vi "Main-dataQ.vi"() -> ()   [LabVIEW 2013]
uses:
  ctl/config_ctl.ctl
  ctl/strain_ctl.ctl
  <vilib>/measure/mascope.llb/Amplitude and Levels 1 chan.vi
  <vilib>/measure/NI_MAPro.lvlib
panel:
  out "error out":errorcluster
  out "원소":enum16{"ini", "grab", "close"}(ring)
  out "grab loop":i32
  out "cam loop":i32
  out "strain loop":i32
  in  "Nulling":bool
  in  "pause":bool
  in  "START":bool
  in  "save_setting":bool
  in  "load_setting":bool
  out "data loop":i32
  out "dt":u32
  in  "Main tap":T1(tab)
  out "right":dbl(slide) scale=0.0..0.5
  out "left":dbl(slide)
  out "rear":dbl(slide) scale=0.0..0.5
  out "front":dbl(slide)
  out "trigger":bool
  out "Triggered Force graph":waveform(dbl)(graph)={"t0"=timestamp(0 s since 1904-01-01), "dt"=0.00062, "Y"=array[3100 elements]}
  out "bonding force":dbl=1.1386680148675508 caption="Bonding force (kg)" format="%.3f"
  out "Bonding time":dbl=0.5053000000000001 format="%.3f"
  out "vacum":dbl=1.2177873383633695 format="%#_3f"
  out "Heater temp":dbl=nan format="%0.2f"
  out "XY 그래프":cluster{dbl[], dbl[]}(graph)
  out "Filtered force 그래프":waveform(dbl)[](graph)
  out "vacuum 차트 3":waveform(dbl)(graph)={"t0"=timestamp(3477442777.176875 s since 1904-01-01), "dt"=0.01, "Y"=[0.9261417940939543, 0.9261417940939543, 0.9261417940939543, 0.9261417940939543, 0.9261417940939543, 0.9261417940939543, 0.9261417940939543, 0.9261417940939543, 0.9261417940939543, 0.9261417940939543], "attributes"=variant("NI_ChannelName"=variant(string "전압"), "NI_UnitDescription"=variant(string "Volts"))}
  out "Force raw chart":waveform(dbl)[](graph)=[{"t0"=timestamp(3477442777.13187 s since 1904-01-01), "dt"=0.00062, "Y"=[-1.6112136636470233e-05, -8.569886798010926e-06, -1.9875060209823524e-07, 2.38297423695265e-06, -2.5658168581669667e-06, -1.772821098699811e-06, -4.127955201515539e-06, 6.359857628775875e-07, 4.928880013384412e-07, -3.030881455329775e-06, -1.6476111269731543e-06, -3.5257574105908386e-06, 3.9272455815972755e-06, 4.1657435117466915e-06, 1.9357923056845556e-06, -8.873963893666015e-06, -7.478785108954976e-06, 2.961286460921625e-07, 1.4110617831093333e-07, -1.8980310390713461e-06, 1.6734457588159683e-06, -1.091306434532689e-05, -1.0513727362142483e-06, -6.190924313818898e-06, -1.2540761368932031e-05, -2.1656959207560037e-05, -7.4907097304474685e-06, -3.2872630354662113e-06, -7.950263527933837e-08, -5.964355867846931e-06, -2.4107952296524134e-06, -3.7881010918357573e-06, 2.609546568115507e-06, 1.715182700246618e-06, -5.290612250873919e-06, -6.512889823589868e-06, -3.120361442334684e-07, 5.578846081749961e-06, 7.045614998740958e-06, -1.4627773018794912e-06, -7.937882831116044e-06, -2.595628704294203e-06, 1.2799261966089874e-06, 3.3190306855961753e-07, -3.4363220332503078e-06, -9.953137975658443e-06, 2.3591245238553327e-06, -1.0871470597100204e-06, 8.685197127258367e-07, -7.478785108954976e-06, -8.659321257106097e-06, -4.879210834785539e-06, -3.710590473067321e-06, -4.771888670569855e-06, -1.2516912366543758e-05, -5.576804340679935e-06, -6.274396873296863e-06, -8.546139112344271e-07, 2.2696881098723825e-06, -3.585380986597095e-06, -7.890184386099151e-06, 4.034519211733817e-07, 2.055040781583931e-06, 3.3071514956147953e-06, -2.7625750097582926e-06, -6.900440625190667e-06, 4.2909549706155075e-06, 9.830102788370948e-06, 3.032879356729265e-06, 4.088231671969834e-06, -9.488079817087242e-06, -5.111742111559042e-06, 2.567809552028929e-06, -4.688415860253707e-06, -1.833603522524735e-05, -9.50012139076079e-07, 3.3250388142463035e-06, -2.6135158111173114e-06, -6.769269618278701e-06, -2.0929577385222132e-05, -7.305878065355784e-06, -1.8562943957647073e-06, -3.090505090348801e-06, -3.5257574105908386e-06, -4.932871908254762e-06, -1.033522309183479e-07, -4.169691655199052e-06, 1.94771715199473e-06, -5.254838228130094e-06, -5.147516144541169e-06, 1.2978134427175586e-06, 9.126526251121246e-06, 1.5422725370008507e-06, -4.688415860253707e-06, -2.005353820147982e-06, 4.4518875659287035e-07, 1.7688444872052448e-06, -1.1229213806461855e-06, -6.51885214588969e-06, -1.4490413466475015e-05], "attributes"=variant("NI_ChannelName"=variant(string "변형률_0"), "NI_UnitDescription"=variant(string "Strain"))}, {"t0"=timestamp(3477442777.13187 s since 1904-01-01), "dt"=0.00062, "Y"=[-1.5926450874775857e-06, 1.7934307923881257e-06, -2.236473822173629e-06, -4.09045749208906e-06, -3.881810155491518e-06, 1.7218937409129746e-06, 3.9872386740088464e-06, 1.7192680555871353e-07, 2.2286147427125606e-06, -1.3005373326004466e-06, 3.456670124526979e-06, 8.523920832607e-06, 5.322604705970085e-06, 3.104945216654824e-06, 2.639953345335169e-06, 6.449322569493326e-06, 1.898110120282012e-07, -2.9306233811443237e-07, -7.929552945691535e-06, 2.53892933758521e-05, 6.6698972632327115e-06, 5.113953528386892e-06, 2.425341858268832e-06, -5.911320745626876e-07, -2.8385721664852527e-06, 1.0303694376600552e-06, -3.2286931975534613e-07, -4.793896442446842e-06, -2.7789585013682837e-06, -2.254357941858881e-06, 4.482039064584e-06, 3.188405341896096e-06, 2.890333530003795e-06, 1.5370897386411374e-06, 1.3224787249476363e-06, 5.0603003825103886e-06, 4.470116157849115e-06, 2.0378491288205883e-06, 3.087060905915481e-06, 4.237619533343155e-06, 6.22874797305966e-06, 2.4551490037417866e-06, 8.455656909807571e-07, -1.976799849226179e-07, -2.862417630541878e-06, 5.030493081733363e-06, 2.8068734545164028e-06, -7.640124402846258e-07, -2.105323591603382e-06, 2.3750223240719277e-07, 6.884510572159387e-06, -7.878580032793122e-07, -5.163499562134611e-06, -6.391533772034915e-06, -2.6835766223972933e-06, 4.684728522578421e-06, 2.885317683250044e-08, -1.2826531787987904e-06, -2.8206880676963555e-06, 3.7726266086577194e-06, 6.7414350226397595e-06, 3.3195569954219583e-06, 2.017338166964026e-07, 2.7114905281608864e-06, 3.40301715648635e-06, 9.60891530636603e-06, -7.029395011258529e-06, 2.153804825353152e-05, 1.1194680695472973e-05, -9.786224662971449e-07, 8.702765913475292e-06, -2.558387878634849e-06, -5.911320745626876e-07, -2.4272377325028147e-06, 2.8307191889483254e-06, 5.656446771208991e-06, 1.9901577367198323e-06, -2.2960875519699664e-06, -4.656785538247539e-06, -2.898185824494624e-06, 7.501831387741804e-07, -3.983153158427838e-06, -1.610529230191517e-06, -2.8028039682679484e-06, 4.458193251398366e-06, 9.171026170763248e-07, 3.748780829304955e-06, 1.9577241432685033e-07, 3.206289656260379e-06, 2.0974633753433343e-06, 7.442217298655735e-07, 6.548006047634227e-07, -1.8489844052503307e-06, 3.7964723891478954e-06, 8.0470009297029e-06, 2.5863004649327575e-06, 1.1674819390124968e-06, 3.150004752252312e-07, 3.188405341896096e-06, 5.7637531966593845e-06], "attributes"=variant("NI_ChannelName"=variant(string "변형률_1"), "NI_UnitDescription"=variant(string "Strain"))}, {"t0"=timestamp(3477442777.13187 s since 1904-01-01), "dt"=0.00062, "Y"=[-9.774144215970737e-06, -5.761376757146625e-06, 5.947220028941115e-07, -3.8056626676763385e-06, -7.275857412313684e-06, 3.1765375395588494e-06, -3.1557437920494864e-06, -3.000717146469372e-06, 7.974506851273759e-07, -1.8618660842482212e-06, -1.4862235419361472e-06, -6.721343374039278e-06, 8.62045556081355e-06, -3.294812422418737e-07, 2.115189123215763e-06, -2.3030966465335333e-06, -5.773301819593379e-06, -1.1940569250260916e-06, -5.171085810533189e-06, -2.538875015539028e-08, 3.6814298472928053e-07, -8.939395837287375e-06, 2.401395215885246e-06, -4.646382161832467e-06, -7.311632490439199e-06, -2.205074690463858e-05, -3.5313850800753163e-06, -4.425767963291082e-06, -3.6148608835335274e-06, -1.677026138378287e-06, -2.5952626153941553e-06, 3.26404755740087e-07, -2.601225184409818e-06, 1.4056372250135049e-06, -1.1753684800069817e-05, -4.914696596438629e-06, 5.808765257422834e-08, 6.318857576908811e-06, 3.9934195965366175e-06, 5.03688401927312e-06, -6.059503232998047e-06, -5.4811377077647035e-06, 1.3937119916306282e-06, -7.055244373975443e-06, 7.318619848217363e-07, -1.718764196644247e-06, 4.814324809771893e-07, -1.0119968136008337e-05, 1.984011385493666e-06, -1.0131893094502119e-05, -1.0251142663796572e-05, -3.865288210289022e-06, -6.06546576070178e-06, -6.995619211769368e-06, 2.1867406310243084e-06, -1.0119968136008337e-05, -8.080796051007461e-06, -1.7962777241804084e-06, -1.2536827790775241e-06, 1.4771886312832808e-06, 2.2284790153078483e-06, -6.190678826058288e-06, -1.7068390374955085e-06, 1.4593007787556523e-06, 5.024958699283277e-06, 2.1927032571370627e-06, 5.589463616211063e-07, -4.831221009990731e-06, -8.959275481128778e-07, 3.421005752440379e-06, 3.987456948949547e-06, -4.205153667407975e-06, -9.674786147839707e-07, -5.212823577128643e-06, -1.6183772832057885e-05, 9.294241431321112e-06, -3.257107342016943e-06, -4.473468338791205e-06, -1.0316729914785664e-05, -1.128265025116678e-05, -1.0650628513704086e-05, -4.65234470638786e-06, -2.362722368329657e-06, -7.230124280525015e-07, 7.139741589589915e-07, -2.326946936105031e-06, -1.5277486145651072e-05, 1.411599841811428e-06, -3.3703959911923048e-06, -5.7852268817560655e-06, 2.17481537901177e-06, 2.5325730631100896e-06, -1.981117625965015e-06, -2.3209843638189005e-06, -2.6191128910294843e-06, 9.047776678219688e-07, -6.514613263977364e-07, -9.495908490762017e-07, 5.470211484321648e-07, -1.2970025127066287e-05], "attributes"=variant("NI_ChannelName"=variant(string "변형률_2"), "NI_UnitDescription"=variant(string "Strain"))}, {"t0"=timestamp(3477442777.13187 s since 1904-01-01), "dt"=0.00062, "Y"=[-7.598292136517871e-06, -3.990960943167142e-06, -3.961148180242939e-06, 8.446924425047726e-07, -3.865747326939833e-06, -6.459578537381319e-07, -5.028556181360945e-07, -4.313044849763774e-07, -2.0352399287900154e-06, -2.1843042998043006e-06, 2.317459299605134e-06, 2.520188680335006e-06, 1.8642998046072807e-06, 3.1998303138911986e-07, -2.3810692014959805e-06, 1.1129194138591358e-07, -3.919410309162601e-06, -4.181762583788524e-06, -2.9177003579997263e-06, -2.887887531081505e-06, 8.147893563887326e-08, -5.910899132064934e-06, 5.841384650575335e-06, -7.771348670609545e-07, -9.965402760758176e-06, -5.064219224553743e-06, -1.0078689889986319e-05, -8.14684269941332e-06, -4.8913055460130025e-06, -2.0292773530250545e-06, -2.5003206193811262e-06, -4.098286874975869e-06, -3.305266946174274e-06, -4.038661360148547e-06, -2.4228072009909966e-06, -2.1366037059148034e-06, -4.217537883299131e-06, -1.2183663865814867e-06, -2.5062831895288145e-06, 1.1725454274867201e-07, 3.9571845882479464e-06, -1.8087543828407676e-07, -4.0803992212742764e-06, -1.2064412154978175e-06, -5.839348772806825e-06, -1.8563626249113895e-06, -5.213282692541838e-06, -3.1800531582297593e-06, -1.8742503581789873e-06, -3.8360372384809986e-07, -4.181762583788524e-06, -6.0420747641119605e-06, -4.050586463682811e-06, -3.531844197032469e-06, -2.3452937705841765e-06, -7.1034036122986465e-06, -1.32569291353597e-06, -1.6953729967054738e-06, -1.7549987909737935e-06, -2.8699998340773e-06, -4.825717583337447e-06, -2.46454519700197e-06, 1.1964865605783791e-06, 3.378708431566748e-07, 2.889871880335409e-06, 2.0908795007679327e-06, -1.0514139655274806e-06, 5.501512595474361e-06, -3.376817668063878e-06, -4.819755040849376e-06, -1.5701588055974375e-06, -5.064219224553743e-06, -8.904240781442745e-07, 4.028736359651292e-06, -4.1996502338637966e-06, -6.918565604118794e-06, -3.996923495538705e-06, -3.3648925484600175e-06, -1.3024146240405366e-05, -8.289942747279497e-06, -7.061666003521132e-06, -5.165582387620764e-06, -6.823165315097408e-06, -1.0633391403086943e-06, -1.9517638616103747e-06, -5.255020455614867e-06, -2.4705077675762867e-06, -1.7491284040547266e-07, -3.1919782822420984e-06, -2.858074702385669e-06, -1.9815767443457687e-06, 2.317459299605134e-06, 3.927371353185168e-06, 3.665014961285459e-06, 2.186281508816372e-06, -1.0096758515535991e-06, -1.5522710614508004e-06, -6.507151727700881e-06, -2.16045400342839e-06, -2.893850096607393e-06], "attributes"=variant("NI_ChannelName"=variant(string "변형률_3"), "NI_UnitDescription"=variant(string "Strain"))}]
  in  "display":bool=TRUE
  out "vacuum 2":dbl=0.9261417940939543 format="%#_3f"
  out "웨이브폼 그래프 2":waveform(dbl)[](graph)
  out "x-y":u32=99
  out "Filtered force 차트":waveform(dbl)[](graph)
  out "Force raw graph":waveform(dbl)[](graph)=[{"t0"=timestamp(3477442777.13187 s since 1904-01-01), "dt"=0.00062, "Y"=[-1.6112136636470233e-05, -8.569886798010926e-06, -1.9875060209823524e-07, 2.38297423695265e-06, -2.5658168581669667e-06, -1.772821098699811e-06, -4.127955201515539e-06, 6.359857628775875e-07, 4.928880013384412e-07, -3.030881455329775e-06, -1.6476111269731543e-06, -3.5257574105908386e-06, 3.9272455815972755e-06, 4.1657435117466915e-06, 1.9357923056845556e-06, -8.873963893666015e-06, -7.478785108954976e-06, 2.961286460921625e-07, 1.4110617831093333e-07, -1.8980310390713461e-06, 1.6734457588159683e-06, -1.091306434532689e-05, -1.0513727362142483e-06, -6.190924313818898e-06, -1.2540761368932031e-05, -2.1656959207560037e-05, -7.4907097304474685e-06, -3.2872630354662113e-06, -7.950263527933837e-08, -5.964355867846931e-06, -2.4107952296524134e-06, -3.7881010918357573e-06, 2.609546568115507e-06, 1.715182700246618e-06, -5.290612250873919e-06, -6.512889823589868e-06, -3.120361442334684e-07, 5.578846081749961e-06, 7.045614998740958e-06, -1.4627773018794912e-06, -7.937882831116044e-06, -2.595628704294203e-06, 1.2799261966089874e-06, 3.3190306855961753e-07, -3.4363220332503078e-06, -9.953137975658443e-06, 2.3591245238553327e-06, -1.0871470597100204e-06, 8.685197127258367e-07, -7.478785108954976e-06, -8.659321257106097e-06, -4.879210834785539e-06, -3.710590473067321e-06, -4.771888670569855e-06, -1.2516912366543758e-05, -5.576804340679935e-06, -6.274396873296863e-06, -8.546139112344271e-07, 2.2696881098723825e-06, -3.585380986597095e-06, -7.890184386099151e-06, 4.034519211733817e-07, 2.055040781583931e-06, 3.3071514956147953e-06, -2.7625750097582926e-06, -6.900440625190667e-06, 4.2909549706155075e-06, 9.830102788370948e-06, 3.032879356729265e-06, 4.088231671969834e-06, -9.488079817087242e-06, -5.111742111559042e-06, 2.567809552028929e-06, -4.688415860253707e-06, -1.833603522524735e-05, -9.50012139076079e-07, 3.3250388142463035e-06, -2.6135158111173114e-06, -6.769269618278701e-06, -2.0929577385222132e-05, -7.305878065355784e-06, -1.8562943957647073e-06, -3.090505090348801e-06, -3.5257574105908386e-06, -4.932871908254762e-06, -1.033522309183479e-07, -4.169691655199052e-06, 1.94771715199473e-06, -5.254838228130094e-06, -5.147516144541169e-06, 1.2978134427175586e-06, 9.126526251121246e-06, 1.5422725370008507e-06, -4.688415860253707e-06, -2.005353820147982e-06, 4.4518875659287035e-07, 1.7688444872052448e-06, -1.1229213806461855e-06, -6.51885214588969e-06, -1.4490413466475015e-05], "attributes"=variant("NI_ChannelName"=variant(string "변형률_0"), "NI_UnitDescription"=variant(string "Strain"))}, {"t0"=timestamp(3477442777.13187 s since 1904-01-01), "dt"=0.00062, "Y"=[-1.5926450874775857e-06, 1.7934307923881257e-06, -2.236473822173629e-06, -4.09045749208906e-06, -3.881810155491518e-06, 1.7218937409129746e-06, 3.9872386740088464e-06, 1.7192680555871353e-07, 2.2286147427125606e-06, -1.3005373326004466e-06, 3.456670124526979e-06, 8.523920832607e-06, 5.322604705970085e-06, 3.104945216654824e-06, 2.639953345335169e-06, 6.449322569493326e-06, 1.898110120282012e-07, -2.9306233811443237e-07, -7.929552945691535e-06, 2.53892933758521e-05, 6.6698972632327115e-06, 5.113953528386892e-06, 2.425341858268832e-06, -5.911320745626876e-07, -2.8385721664852527e-06, 1.0303694376600552e-06, -3.2286931975534613e-07, -4.793896442446842e-06, -2.7789585013682837e-06, -2.254357941858881e-06, 4.482039064584e-06, 3.188405341896096e-06, 2.890333530003795e-06, 1.5370897386411374e-06, 1.3224787249476363e-06, 5.0603003825103886e-06, 4.470116157849115e-06, 2.0378491288205883e-06, 3.087060905915481e-06, 4.237619533343155e-06, 6.22874797305966e-06, 2.4551490037417866e-06, 8.455656909807571e-07, -1.976799849226179e-07, -2.862417630541878e-06, 5.030493081733363e-06, 2.8068734545164028e-06, -7.640124402846258e-07, -2.105323591603382e-06, 2.3750223240719277e-07, 6.884510572159387e-06, -7.878580032793122e-07, -5.163499562134611e-06, -6.391533772034915e-06, -2.6835766223972933e-06, 4.684728522578421e-06, 2.885317683250044e-08, -1.2826531787987904e-06, -2.8206880676963555e-06, 3.7726266086577194e-06, 6.7414350226397595e-06, 3.3195569954219583e-06, 2.017338166964026e-07, 2.7114905281608864e-06, 3.40301715648635e-06, 9.60891530636603e-06, -7.029395011258529e-06, 2.153804825353152e-05, 1.1194680695472973e-05, -9.786224662971449e-07, 8.702765913475292e-06, -2.558387878634849e-06, -5.911320745626876e-07, -2.4272377325028147e-06, 2.8307191889483254e-06, 5.656446771208991e-06, 1.9901577367198323e-06, -2.2960875519699664e-06, -4.656785538247539e-06, -2.898185824494624e-06, 7.501831387741804e-07, -3.983153158427838e-06, -1.610529230191517e-06, -2.8028039682679484e-06, 4.458193251398366e-06, 9.171026170763248e-07, 3.748780829304955e-06, 1.9577241432685033e-07, 3.206289656260379e-06, 2.0974633753433343e-06, 7.442217298655735e-07, 6.548006047634227e-07, -1.8489844052503307e-06, 3.7964723891478954e-06, 8.0470009297029e-06, 2.5863004649327575e-06, 1.1674819390124968e-06, 3.150004752252312e-07, 3.188405341896096e-06, 5.7637531966593845e-06], "attributes"=variant("NI_ChannelName"=variant(string "변형률_1"), "NI_UnitDescription"=variant(string "Strain"))}, {"t0"=timestamp(3477442777.13187 s since 1904-01-01), "dt"=0.00062, "Y"=[-9.774144215970737e-06, -5.761376757146625e-06, 5.947220028941115e-07, -3.8056626676763385e-06, -7.275857412313684e-06, 3.1765375395588494e-06, -3.1557437920494864e-06, -3.000717146469372e-06, 7.974506851273759e-07, -1.8618660842482212e-06, -1.4862235419361472e-06, -6.721343374039278e-06, 8.62045556081355e-06, -3.294812422418737e-07, 2.115189123215763e-06, -2.3030966465335333e-06, -5.773301819593379e-06, -1.1940569250260916e-06, -5.171085810533189e-06, -2.538875015539028e-08, 3.6814298472928053e-07, -8.939395837287375e-06, 2.401395215885246e-06, -4.646382161832467e-06, -7.311632490439199e-06, -2.205074690463858e-05, -3.5313850800753163e-06, -4.425767963291082e-06, -3.6148608835335274e-06, -1.677026138378287e-06, -2.5952626153941553e-06, 3.26404755740087e-07, -2.601225184409818e-06, 1.4056372250135049e-06, -1.1753684800069817e-05, -4.914696596438629e-06, 5.808765257422834e-08, 6.318857576908811e-06, 3.9934195965366175e-06, 5.03688401927312e-06, -6.059503232998047e-06, -5.4811377077647035e-06, 1.3937119916306282e-06, -7.055244373975443e-06, 7.318619848217363e-07, -1.718764196644247e-06, 4.814324809771893e-07, -1.0119968136008337e-05, 1.984011385493666e-06, -1.0131893094502119e-05, -1.0251142663796572e-05, -3.865288210289022e-06, -6.06546576070178e-06, -6.995619211769368e-06, 2.1867406310243084e-06, -1.0119968136008337e-05, -8.080796051007461e-06, -1.7962777241804084e-06, -1.2536827790775241e-06, 1.4771886312832808e-06, 2.2284790153078483e-06, -6.190678826058288e-06, -1.7068390374955085e-06, 1.4593007787556523e-06, 5.024958699283277e-06, 2.1927032571370627e-06, 5.589463616211063e-07, -4.831221009990731e-06, -8.959275481128778e-07, 3.421005752440379e-06, 3.987456948949547e-06, -4.205153667407975e-06, -9.674786147839707e-07, -5.212823577128643e-06, -1.6183772832057885e-05, 9.294241431321112e-06, -3.257107342016943e-06, -4.473468338791205e-06, -1.0316729914785664e-05, -1.128265025116678e-05, -1.0650628513704086e-05, -4.65234470638786e-06, -2.362722368329657e-06, -7.230124280525015e-07, 7.139741589589915e-07, -2.326946936105031e-06, -1.5277486145651072e-05, 1.411599841811428e-06, -3.3703959911923048e-06, -5.7852268817560655e-06, 2.17481537901177e-06, 2.5325730631100896e-06, -1.981117625965015e-06, -2.3209843638189005e-06, -2.6191128910294843e-06, 9.047776678219688e-07, -6.514613263977364e-07, -9.495908490762017e-07, 5.470211484321648e-07, -1.2970025127066287e-05], "attributes"=variant("NI_ChannelName"=variant(string "변형률_2"), "NI_UnitDescription"=variant(string "Strain"))}, {"t0"=timestamp(3477442777.13187 s since 1904-01-01), "dt"=0.00062, "Y"=[-7.598292136517871e-06, -3.990960943167142e-06, -3.961148180242939e-06, 8.446924425047726e-07, -3.865747326939833e-06, -6.459578537381319e-07, -5.028556181360945e-07, -4.313044849763774e-07, -2.0352399287900154e-06, -2.1843042998043006e-06, 2.317459299605134e-06, 2.520188680335006e-06, 1.8642998046072807e-06, 3.1998303138911986e-07, -2.3810692014959805e-06, 1.1129194138591358e-07, -3.919410309162601e-06, -4.181762583788524e-06, -2.9177003579997263e-06, -2.887887531081505e-06, 8.147893563887326e-08, -5.910899132064934e-06, 5.841384650575335e-06, -7.771348670609545e-07, -9.965402760758176e-06, -5.064219224553743e-06, -1.0078689889986319e-05, -8.14684269941332e-06, -4.8913055460130025e-06, -2.0292773530250545e-06, -2.5003206193811262e-06, -4.098286874975869e-06, -3.305266946174274e-06, -4.038661360148547e-06, -2.4228072009909966e-06, -2.1366037059148034e-06, -4.217537883299131e-06, -1.2183663865814867e-06, -2.5062831895288145e-06, 1.1725454274867201e-07, 3.9571845882479464e-06, -1.8087543828407676e-07, -4.0803992212742764e-06, -1.2064412154978175e-06, -5.839348772806825e-06, -1.8563626249113895e-06, -5.213282692541838e-06, -3.1800531582297593e-06, -1.8742503581789873e-06, -3.8360372384809986e-07, -4.181762583788524e-06, -6.0420747641119605e-06, -4.050586463682811e-06, -3.531844197032469e-06, -2.3452937705841765e-06, -7.1034036122986465e-06, -1.32569291353597e-06, -1.6953729967054738e-06, -1.7549987909737935e-06, -2.8699998340773e-06, -4.825717583337447e-06, -2.46454519700197e-06, 1.1964865605783791e-06, 3.378708431566748e-07, 2.889871880335409e-06, 2.0908795007679327e-06, -1.0514139655274806e-06, 5.501512595474361e-06, -3.376817668063878e-06, -4.819755040849376e-06, -1.5701588055974375e-06, -5.064219224553743e-06, -8.904240781442745e-07, 4.028736359651292e-06, -4.1996502338637966e-06, -6.918565604118794e-06, -3.996923495538705e-06, -3.3648925484600175e-06, -1.3024146240405366e-05, -8.289942747279497e-06, -7.061666003521132e-06, -5.165582387620764e-06, -6.823165315097408e-06, -1.0633391403086943e-06, -1.9517638616103747e-06, -5.255020455614867e-06, -2.4705077675762867e-06, -1.7491284040547266e-07, -3.1919782822420984e-06, -2.858074702385669e-06, -1.9815767443457687e-06, 2.317459299605134e-06, 3.927371353185168e-06, 3.665014961285459e-06, 2.186281508816372e-06, -1.0096758515535991e-06, -1.5522710614508004e-06, -6.507151727700881e-06, -2.16045400342839e-06, -2.893850096607393e-06], "attributes"=variant("NI_ChannelName"=variant(string "변형률_3"), "NI_UnitDescription"=variant(string "Strain"))}]
  out "강도 그래프 2":dbl[][](graph)=[[nan, nan, nan, nan], [nan, nan, nan, nan]]
  out "Image":T2(plugin-control)
  out "Heater temp 2":dbl=nan caption="Heater temp" format="%0.2f"
  in  "Config":T3={"Trigger minlevel"=0.5, "Lower Cut-Off"=20.0, "Force high_level"=0.0, "state settings"={"method"=enum."histogram", "histogram size"=512, "histogram method"=enum."mode", "reserved"=1.0}} {"state settings"."reserved" format="%0.2f"; "Trigger minlevel" format="%#_13g"}
  out "offset":T4
  in  "정지":bool=TRUE
  # "Die Attach Machine Monitoring"
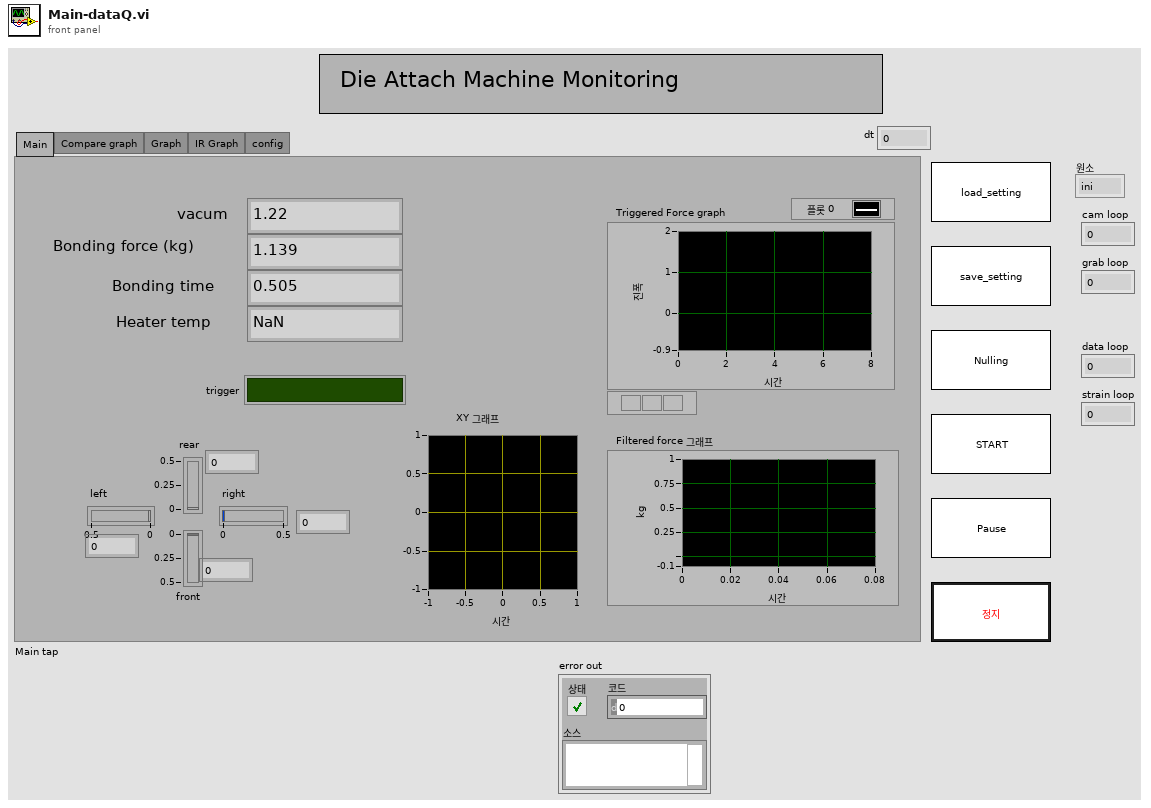
[diagram p1: front panel]
types:
  T1 = enum32{"Main", "Compare graph", "Graph", "IR Graph", "config"}
  T2 = typedef "IMAQ Image.ctl" = refnum<image>
  T3 = typedef "config_ctl.ctl" = cluster{"Trigger minlevel":dbl, "Lower Cut-Off":dbl, "Force high_level":dbl, "state settings":cluster{"method":enum32{"histogram", "peak", "auto select"}, "histogram size":i32, "histogram method":enum16{"mode"}, "reserved":dbl}}
  T4 = cluster{"DC value":dbl, "DC value":dbl, "DC value":dbl, "DC value":dbl}
  T5 = enum32{"Main", "Compare graph", "Graph", "IR Graph", "config", "offset val"}
  T6 = cluster{"Global Rectangle":i32[], "Contours":cluster{"Contour Type":u32, "ROI Type":u32, "Points":i32[]}[]}
  T7 = typedef "strain_ctl.ctl" = enum16{"config", "start", "read", "close"}
  T8 = cluster{"high state level":dbl, "high state level":dbl, "high state level":dbl, "high state level":dbl}
  T9 = cluster{"method":enum32{"histogram", "peak", "auto select"}, "histogram size":i32, "histogram method":enum16{"mode"}, "reserved":dbl}
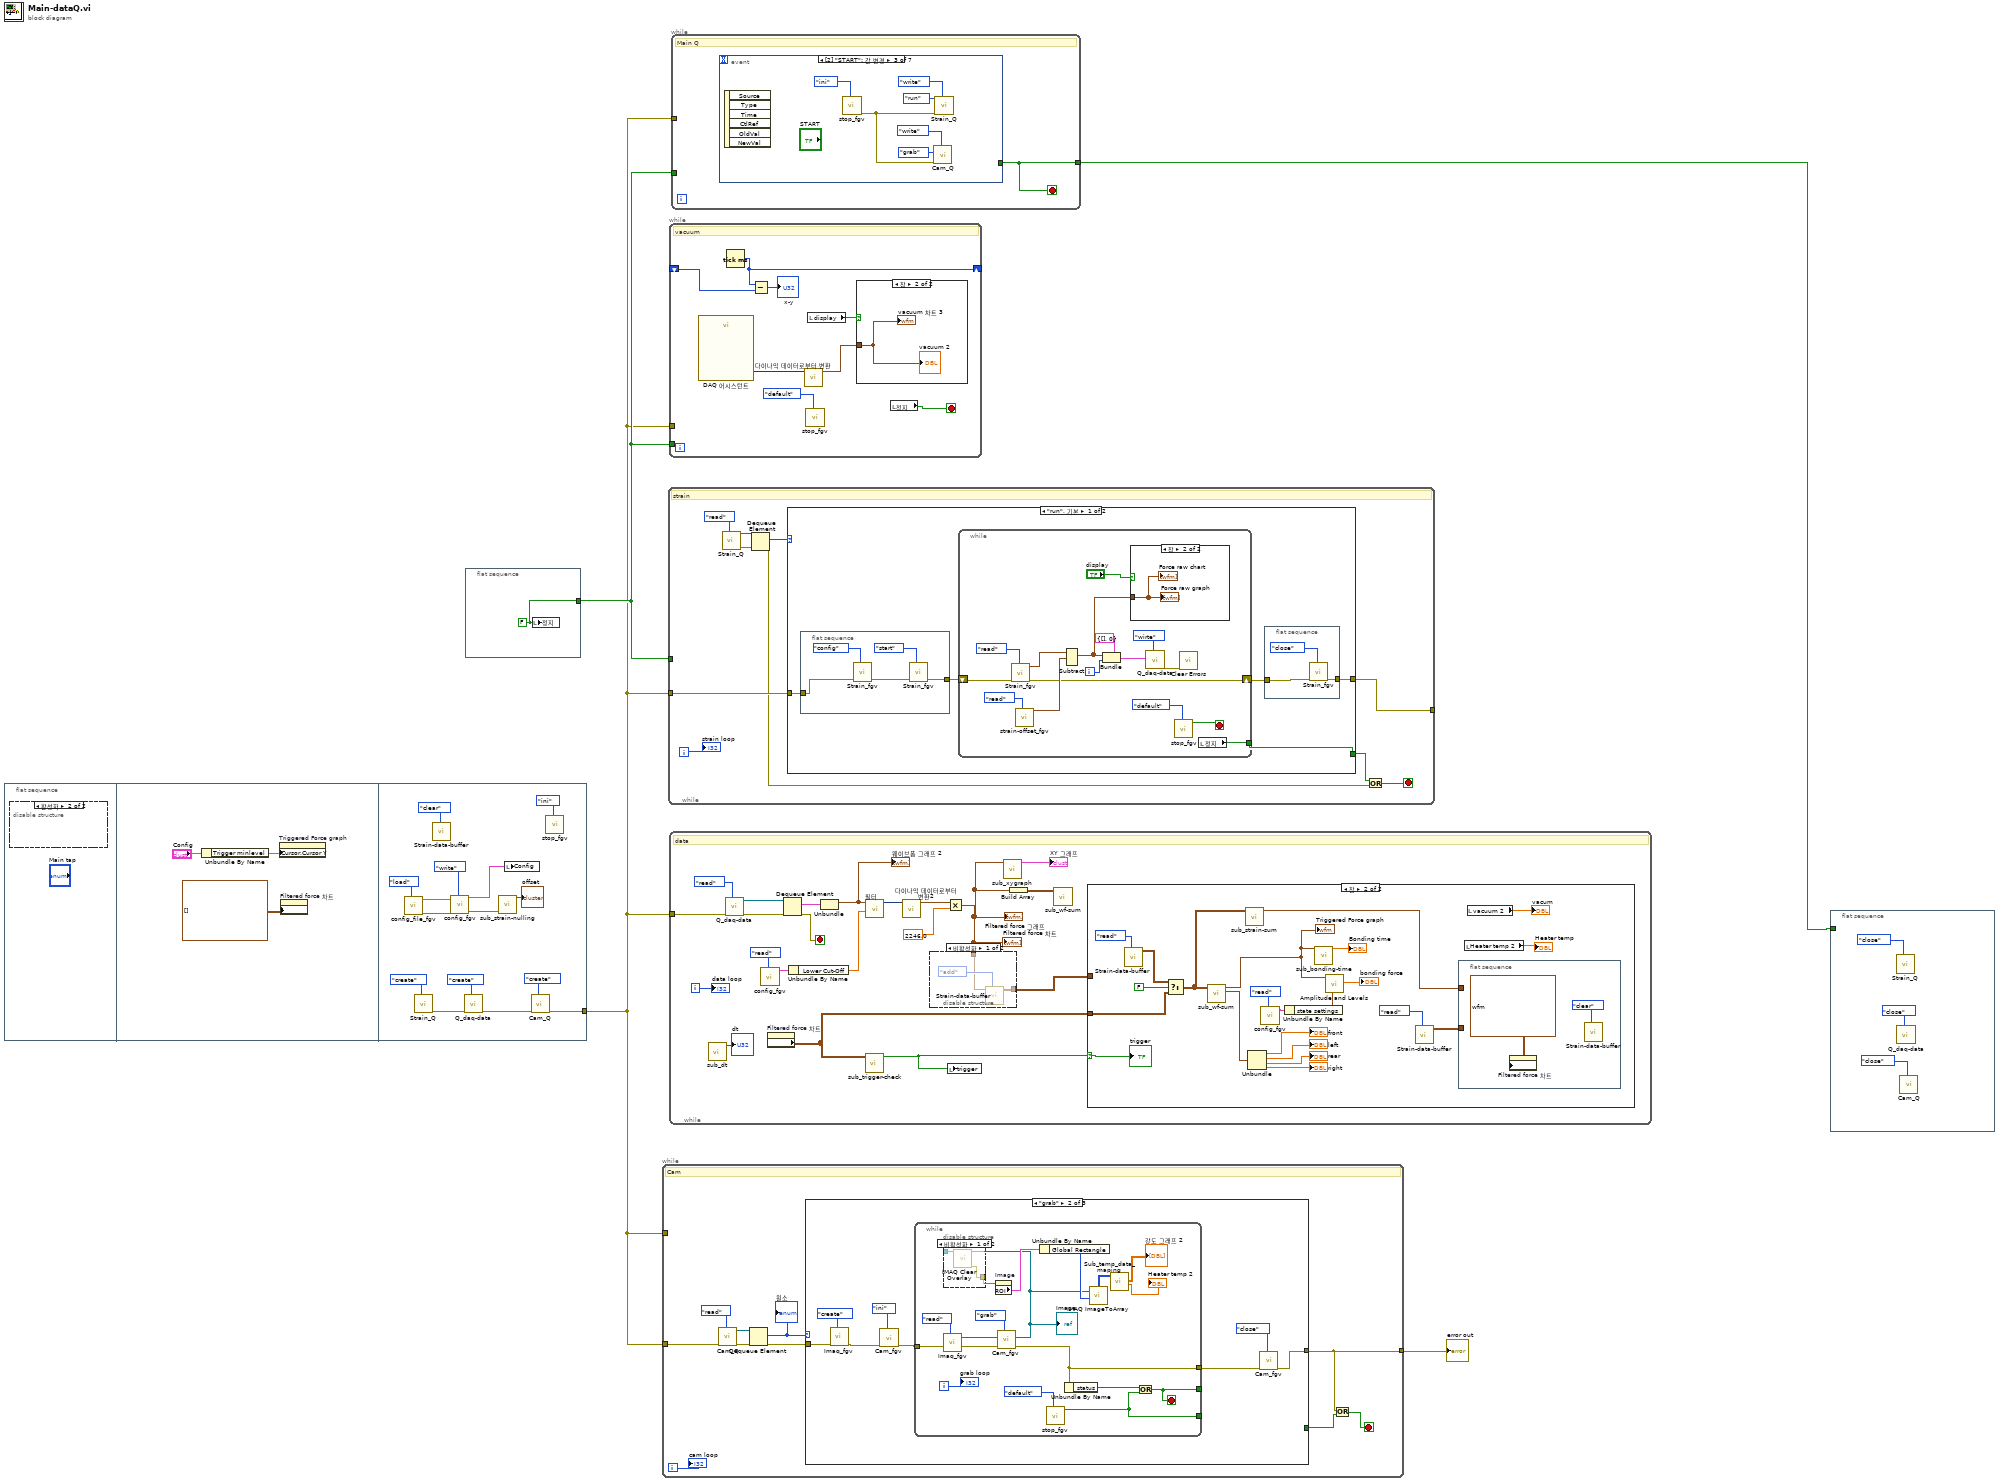
[diagram p0: block diagram]
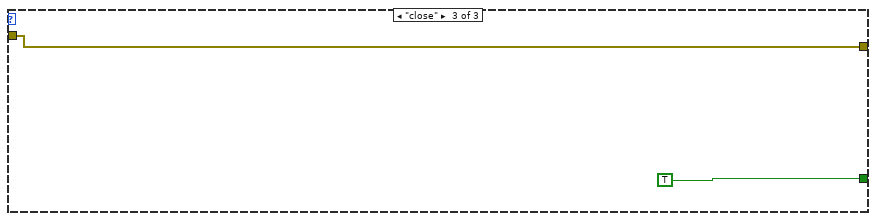
[diagram p4: hidden frame]
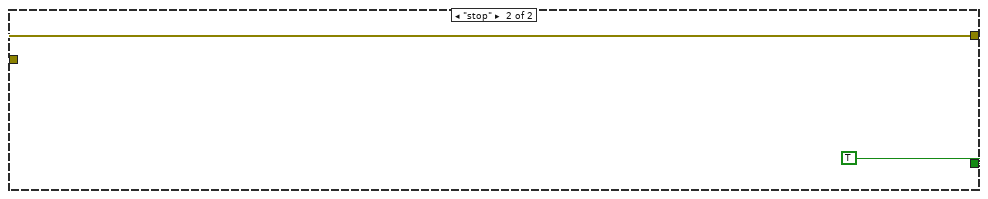
[diagram p6: hidden frame]
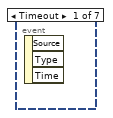
[diagram p7: hidden frame]
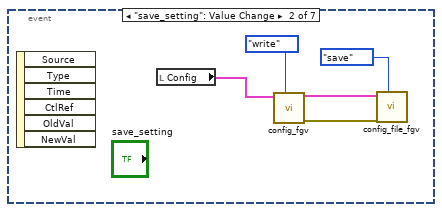
[diagram p8: hidden frame]
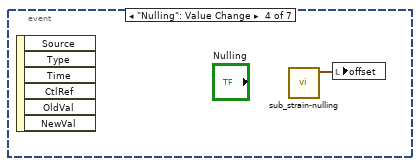
[diagram p9: hidden frame]
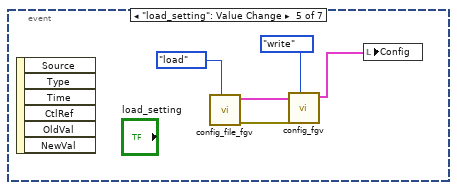
[diagram p10: hidden frame]
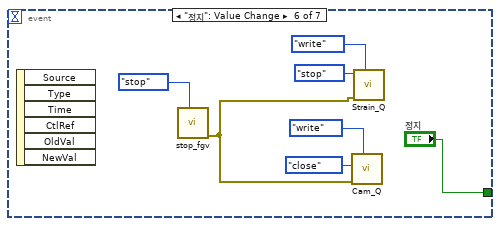
[diagram p11: hidden frame]
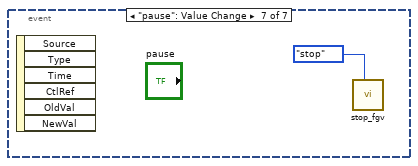
[diagram p12: hidden frame]
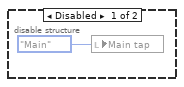
[diagram p13: hidden frame]
diagram:
  n1 = flat-sequence {
    tunnel: [w18] -> w2
    frame #0 {
      n2 = disable-structure shown="활성화" {
        frame Disabled {
          n3 = local write "Main tap"(T5."Main" ("Main tap")) -> ()
        }
        frame Enabled {
        }
      }
    }
    frame #1 {
      n4 = Unbundle By Name("Config") -> ("Trigger minlevel"=w7:dbl)
      n5 = property on="Triggered Force graph" class="WFGraph (엄격한)"("Cursor.Cursor Y"=w7) -> ()  [unwired: 2 in, 2 out]
      n6 = property on="Filtered force 차트" class="WFChart (엄격한)"("History Data"=waveform(dbl)[][] [] ("히스토리 데이터")) -> ()  [unwired: 2 in, 2 out]
    }
    frame #2 {
      n7 = call "config_file_fgv.vi"("cmd"=enum16{"save", "load"}."load") -> ("error out"=w13:errorcluster, "var"=w14:T3)  [unwired: 8 in, 1 out]
      n8 = call "Strain_Q.vi"("cmd"=enum16{"create", "write", "read", "close"}."create") -> ("error out"=w21:errorcluster)  [unwired: 9 in, 1 out]
      n9 = call "Strain-data-buffer.vi"("cmd"=enum16{"clear", "add", "read"}."clear") -> ()  [unwired: 10 in, 1 out]
      n10 = call "config_fgv.vi"("cmd"=enum16{"write", "read", "ini"}."write", "error in (no error)"=w13, "Config in"=w14) -> ("error out"=w9:errorcluster, "Config out"=w15:T3)  [unwired: 7 in]
      n11 = call "Q_daq-data.vi"("cmd"=enum16{"create", "wirte", "read", "close"}."create", "error in"=w21) -> ("error out"=w19:errorcluster)  [unwired: 8 in, 1 out]
      n12 = call "sub_strain-nulling.vi"("error in"=w9) -> ("offset"=→"offset":T4)  [unwired: 9 in, 1 out]
      n13 = local write "Config"(w15) -> ()
      n14 = call "Cam_Q.vi"("cmd"=enum16{"create", "write", "read", "close"}."create", "error in"=w19) -> ("error out"=w18:errorcluster)  [unwired: 8 in, 1 out]
      n15 = call "stop_fgv.vi"("cmd"=enum16{"default", "ini", "stop"}."ini") -> ()  [unwired: 9 in, 2 out]
    }
  }
  n16 = flat-sequence {
    tunnel: [w24] -> w4
    frame #0 {
      w24 = FALSE ("정지")
      n17 = local write "정지"(w24) -> ()
    }
  }
  n18 = while {
    tunnel: w2 -> [_]
    tunnel: [w26] -> w1
    tunnel: w2 -> [w28]
    i -> [w31]
    stop <- w25 stop-if-true
    # "Cam"
    n19 = call "Cam_Q.vi"("cmd"=enum16{"create", "write", "read", "close"}."read", "error in"=w28) -> ("error out"=w33:errorcluster, "queue out"=w32:refnum<queue>)  [unwired: 8 in]
    n20 = Dequeue Element(queue=w32, error in (no error)=w33) -> (element=w29:enum16{"ini", "grab", "close"}, error out=w30:errorcluster)  [unwired: 1 in, 2 out]
    "원소" <- w29
    n21 = case shown="\"grab\"" w29 {
      tunnel: w30 -> [w35 w40 w63]
      tunnel: [_ _ TRUE ("정지")] -> w27
      tunnel: [w35 w36 w63] -> w26
      frame "ini", Default {
      }
      frame "grab" {
        n22 = call "Imaq_fgv.vi"("cmd"=enum16{"create", "close", "read"}."create", "error in"=w40) -> ("error out"=w43:errorcluster)  [unwired: 8 in, 1 out]
        n23 = call "Cam_fgv.vi"("cmd"=enum16{"ini", "grab", "close"}."ini", "error in"=w43) -> ("error out"=w39:errorcluster)  [unwired: 8 in, 1 out]
        n24 = while {
          tunnel: w39 -> [w52]
          tunnel: [w51] -> w37
          tunnel: [w55] -> _
          tunnel: [w44] -> _
          i -> [w46]
          stop <- w55 stop-if-true
          n25 = call "Imaq_fgv.vi"("cmd"=enum16{"create", "close", "read"}."read") -> ("New Image"=w49:T2)  [unwired: 9 in, 1 out]
          n26 = call "Cam_fgv.vi"("cmd"=enum16{"ini", "grab", "close"}."grab", "error in"=w52, "Image In"=w49) -> ("error out"=w51:errorcluster, "Image Out"=w53:T2)  [unwired: 7 in]
          "Image" <- w53
          n27 = disable-structure shown="비활성화" {
            disable-tunnel: w53 -> [w62 _]
            disable-tunnel: [w61 _] -> w59
            frame Disabled {
              n28 = call "IMAQ Clear Overlay"("Image"=w62) -> ("error out"=w61:errorcluster)  [unwired: 9 in, 1 out]
            }
            frame Enabled {
            }
          }
          n29 = property on="Image" class="ImageControl"(error in=w59) -> ("ROI"=w58:T6)  [unwired: 1 in, 2 out]
          n30 = Unbundle By Name(w58) -> ("Global Rectangle"=w57:i32[])
          n31 = call "stop_fgv.vi"("cmd"=enum16{"default", "ini", "stop"}."default") -> ("stop"=w44:bool)  [unwired: 9 in, 1 out]
          n32 = Unbundle By Name(w51) -> ("status"=w60:bool)
          n33 = call "IMAQ ImageToArray"("Optional Rectangle"=w57, "Image"=w53) -> ("Image Pixels (U8)"=w56:u8[][])  [unwired: 2 in, 4 out]
          n34 = call "Sub_temp_data_maping.vi"("temp_data"=w56) -> ("mean"=→"Heater temp 2":dbl, "intensity"=→"강도 그래프 2":dbl[][])  [unwired: 8 in, 1 out]
          n35 = Or(x=w60, y=w44) -> (x .or. y?=w55:bool)
          "grab loop" <- w46
        }
        n36 = call "Cam_fgv.vi"("cmd"=enum16{"ini", "grab", "close"}."close", "error in"=w37) -> ("error out"=w36:errorcluster)  [unwired: 8 in, 1 out]
      }
      frame "close" {
      }
    }
    n37 = Or(x=w26, y=w27) -> (x .or. y?=w25:bool)
    "cam loop" <- w31
  }
  "error out" <- w1
  n38 = while {
    tunnel: [w74] -> _
    tunnel: w4 -> [_]
    tunnel: w2 -> [w73]
    i -> [w68]
    stop <- w65 stop-if-true
    # "strain"
    n39 = call "Strain_Q.vi"("cmd"=enum16{"create", "write", "read", "close"}."read") -> ("error out"=w71:errorcluster, "queue out"=w70:refnum<queue>)  [unwired: 9 in]
    n40 = Dequeue Element(queue=w70, error in (no error)=w71) -> (element=w69:enum16{"run", "stop", "close"}, error out=w66:errorcluster)  [unwired: 1 in, 2 out]
    n41 = case shown="\"run\", 기본" w69 {
      tunnel: [w77 w106] -> w74
      tunnel: w73 -> [w76 w106]
      tunnel: [w75 TRUE ("정지")] -> w67
      frame "run", Default {
        n42 = flat-sequence {
          tunnel: [w83] -> w78
          tunnel: w76 -> [w86]
          frame #0 {
            n43 = call "Strain_fgv.vi"("cmd"=strain_ctl."config", "error in"=w86) -> ("error out"=w84:errorcluster)  [unwired: 8 in, 1 out]
            n44 = call "Strain_fgv.vi"("cmd"=strain_ctl."start", "error in"=w84) -> ("error out"=w83:errorcluster)  [unwired: 8 in, 1 out]
          }
        }
        n45 = while {
          tunnel: [w89] -> w75
          shift-right: [w90] -> w79
          shift-left: w78 -> [w92]
          i -> [w102]
          stop <- w94 stop-if-true
          n46 = call "Strain_fgv.vi"("cmd"=strain_ctl."read", "error in"=w92) -> ("error out"=w90:errorcluster, "data"=w91:waveform(dbl)[])  [unwired: 8 in]
          n47 = call "strain-offset_fgv.vi"("열거형"=enum16{"write", "read"}."read") -> ("Strain_offset_data"=w99:waveform(dbl)[])  [unwired: 10 in]
          n48 = Subtract(1:w99, 2:w91) -> (0:w98:waveform(dbl)[])  [unwired: 1 in, 1 out]
          n49 = Bundle(cluster=cluster{"data":waveform(dbl)[], i32} {"data"=[], 0}, "data"=w98, w102) -> (w96:cluster{"data":waveform(dbl)[], i32})
          n50 = case shown="참" "display" {
            tunnel: w98 -> [_ w104]
            frame False {
            }
            frame True {
              "Force raw graph" <- w104
              "Force raw chart" <- w104
            }
          }
          n51 = call "Q_daq-data.vi"("cmd"=enum16{"create", "wirte", "read", "close"}."wirte", "data"=w96) -> ("error out"=w88:errorcluster)  [unwired: 8 in, 1 out]
          n52 = call "stop_fgv.vi"("cmd"=enum16{"default", "ini", "stop"}."default") -> ("stop"=w94:bool)  [unwired: 9 in, 1 out]
          n53 = call <vilib>:"Clear Errors.vi"("error in (no error)"=w88) -> ()  [unwired: 6 in, 1 out]
          n54 = local read "정지"() -> (w89:bool)
        }
        n55 = flat-sequence {
          tunnel: w79 -> [w81]
          tunnel: [w80] -> w77
          frame #0 {
            n56 = call "Strain_fgv.vi"("cmd"=strain_ctl."close", "error in"=w81) -> ("error out"=w80:errorcluster)  [unwired: 8 in, 1 out]
          }
        }
      }
      frame "stop" {
      }
    }
    n57 = Or(x=w67, y=w66) -> (x .or. y?=w65:bool)
    "strain loop" <- w68
  }
  n58 = while {
    tunnel: w4 -> [_]
    shift-right: [w114] -> _
    shift-left: _ -> [w113]
    tunnel: w2 -> [_]
    stop <- w107 stop-if-true
    # "vacuum"
    n59 = call "DAQ 어시스턴트"() -> ("data"=w111:dynamicdata)  [unwired: 16 in, 3 out]
    n60 = Tick Count (ms)() -> (millisecond timer value=w114:u32)
    n61 = Subtract(x=w114, y=w113) -> (x-y=→"x-y":u32)
    n62 = call "다이나믹 데이터로부터 변환"("Dynamic Data Type"=w111) -> ("Waveform"=w110:waveform(dbl))  [unwired: 3 in]
    n63 = call "stop_fgv.vi"("cmd"=enum16{"default", "ini", "stop"}."default") -> ()  [unwired: 9 in, 2 out]
    n64 = local read "display"() -> (w109:bool)
    n65 = case shown="참" w109 {
      tunnel: w110 -> [_ w115]
      frame False {
      }
      frame True {
        "vacuum 차트 3" <- w115
        "vacuum 2" <- w115
      }
    }
    n66 = local read "정지"() -> (w107:bool)
  }
  n67 = while {
    tunnel: w2 -> [w117]
    i -> [w129]
    stop <- w136 stop-if-true
    # "data"
    n68 = call "sub_dt.vi"() -> ("dt"=→"dt":u32)  [unwired: 11 in]
    n69 = call "Q_daq-data.vi"("cmd"=enum16{"create", "wirte", "read", "close"}."read", "error in"=w117) -> ("error out"=w116:errorcluster, "queue out"=w118:refnum<queue>)  [unwired: 8 in]
    n70 = call "config_fgv.vi"("cmd"=enum16{"write", "read", "ini"}."read") -> ("Config out"=w125:T3)  [unwired: 9 in, 1 out]
    n71 = property on="Filtered force 차트" class="WFChart (엄격한)"() -> ("History Data"=w124:waveform(dbl)[][])  [unwired: 2 in, 2 out]
    n72 = Dequeue Element(queue=w118, error in (no error)=w116) -> (element=w134:cluster{"data":waveform(dbl)[], i32}, error out=w136:errorcluster)  [unwired: 1 in, 2 out]
    n73 = Unbundle By Name(w125) -> ("Lower Cut-Off"=w127:dbl)
    n74 = Unbundle(w134) -> ("data"=w122:waveform(dbl)[])  [unwired: 1 out]
    "웨이브폼 그래프 2" <- w122
    n75 = call "sub_trigger-check.vi"("wf history"=w124) -> ("stop triiger"=w123:bool)  [unwired: 10 in]
    n76 = call "필터"("Lower Cut-Off"=w127, "Signal"=w122) -> ("Filtered Signal"=w133:dynamicdata)  [unwired: 8 in, 1 out]
    n77 = call "다이나믹 데이터로부터 변환2"("Dynamic Data Type"=w133) -> ("Array of Waveform"=w132:waveform(dbl)[])  [unwired: 3 in]
    n78 = Multiply(x=w132, y=2246.0) -> (x*y=w121:waveform(dbl)[])
    "Filtered force 그래프" <- w121
    "Filtered force 차트" <- w121
    n79 = disable-structure shown="비활성화" {
      disable-tunnel: w121 -> [w138 _]
      disable-tunnel: [w137 _] -> w130
      frame Disabled {
        n80 = call "Strain-data-buffer.vi"("cmd"=enum16{"clear", "add", "read"}."add", "History Data"=w138) -> ("히스토리 데이터 out"=w137:waveform(dbl)[][])  [unwired: 9 in]
      }
      frame Enabled {
      }
    }
    n81 = local write "trigger"(w123) -> ()
    n82 = call "sub_xygraph.vi"("wf"=w121) -> ("클러스터"=→"XY 그래프":cluster{dbl[], dbl[]})  [unwired: 10 in]
    n83 = Build Array(w121) -> (w120:waveform(dbl)[][])
    n84 = call "sub_wf-sum.vi"("History Data"=w120) -> ()  [unwired: 9 in, 2 out]
    n85 = case shown="참" w123 {
      selector: w123 -> [_ w159]
      tunnel: w124 -> [_ w151]
      tunnel: w130 -> [_ _]
      frame False {
      }
      frame True {
        n86 = call "Strain-data-buffer.vi"("cmd"=enum16{"clear", "add", "read"}."read") -> ("히스토리 데이터 out"=w150:waveform(dbl)[][])  [unwired: 10 in]
        n87 = Select(t=w150, s=FALSE, f=w151) -> (s? t:f=w149:waveform(dbl)[][])
        n88 = call "sub_wf-sum.vi"("History Data"=w149) -> ("high level x4"=w145:T8, "sum of wf"=w152:waveform(dbl))  [unwired: 9 in]
        "Triggered Force graph" <- w152
        n89 = call "sub_strain-sum.vi"("waveform history"=w149) -> ("원소 출력"=w140:waveform(dbl))  [unwired: 10 in]
        n90 = Unbundle(w145) -> ("high state level"=→"front":dbl, "high state level"=→"left":dbl, "high state level"=→"rear":dbl, "high state level"=→"right":dbl)
        n91 = call "config_fgv.vi"("cmd"=enum16{"write", "read", "ini"}."read") -> ("Config out"=w147:T3)  [unwired: 9 in, 1 out]
        n92 = Unbundle By Name(w147) -> ("state settings"=w146:T9)
        n93 = call "sub_bonding-time.vi"("원소"=w152) -> ("dt"=→"Bonding time":dbl)  [unwired: 9 in, 1 out]
        n94 = call-poly <vilib>:"Amplitude and Levels.vi"("state settings"=w146, "signal in"=w152) -> ("high state level"=→"bonding force":dbl)  [unwired: 6 in, 3 out]
        n95 = call "Strain-data-buffer.vi"("cmd"=enum16{"clear", "add", "read"}."read") -> ("히스토리 데이터 out"=w155:waveform(dbl)[][])  [unwired: 10 in]
        n96 = flat-sequence {
          tunnel: w155 -> [_]
          tunnel: w140 -> [_]
          frame #0 {
            n97 = property on="Filtered force 차트" class="WFChart (엄격한)"("History Data"=waveform(dbl)[][] [[{"t0"=timestamp(0 s since 1904-01-01), "dt"=0.00062, "Y"=[]}]] ("히스토리 데이터")) -> ()  [unwired: 2 in, 2 out]
            n98 = call "Strain-data-buffer.vi"("cmd"=enum16{"clear", "add", "read"}."clear") -> ()  [unwired: 10 in, 1 out]
          }
        }
        n99 = local read "Heater temp 2"() -> (→"Heater temp":dbl)
        n100 = local read "vacuum 2"() -> (→"vacum":dbl)
        "trigger" <- w159
      }
    }
    "data loop" <- w129
  }
  n101 = while {
    tunnel: w4 -> [_]
    tunnel: [w164] -> w3
    tunnel: w2 -> [_]
    stop <- w164 stop-if-true
    # "Main Q"
    n102 = event shown="[2] \"START\": 값 변경" {
      selector: _ -> [_ _ _ _ _ _ _]
      dyn-events: _ -> [_ _ _ _ _ _ _]
      timeout: _ -> [_ _ _ _ _ _ _]
      tunnel: [_ _ _ _ _ "정지" _] -> w164
      event Timeout {
        n103 = event-data() -> ()  [unwired: 1 in, 3 out]
      }
      event "save_setting": Value Change {
        n104 = event-data() -> ()  [unwired: 1 in, 6 out]
        n105 = local read "Config"() -> (w165:T3)
        n106 = call "config_fgv.vi"("cmd"=enum16{"write", "read", "ini"}."write", "Config in"=w165) -> ("error out"=w167:errorcluster, "Config out"=w166:T3)  [unwired: 8 in]
        n107 = call "config_file_fgv.vi"("cmd"=enum16{"save", "load"}."save", "error in"=w167, "Config"=w166) -> ()  [unwired: 6 in, 3 out]
      }
      event "START": Value Change {
        n108 = event-data() -> ()  [unwired: 1 in, 6 out]
        n109 = call "stop_fgv.vi"("cmd"=enum16{"default", "ini", "stop"}."ini") -> ("error out"=w170:errorcluster)  [unwired: 9 in, 1 out]
        n110 = call "Cam_Q.vi"("cmd"=enum16{"create", "write", "read", "close"}."write", "error in"=w170, "data"=enum16{"ini", "grab", "close"}."grab") -> ()  [unwired: 7 in, 2 out]
        n111 = call "Strain_Q.vi"("cmd"=enum16{"create", "write", "read", "close"}."write", "error in"=w170, "data"=enum16{"run", "stop", "close"}."run") -> ()  [unwired: 7 in, 2 out]
      }
      event "Nulling": Value Change {
        n112 = event-data() -> ()  [unwired: 1 in, 6 out]
        n113 = call "sub_strain-nulling.vi"() -> ("offset"=w176:T4)  [unwired: 10 in, 1 out]
        n114 = local write "offset"(w176) -> ()
      }
      event "load_setting": Value Change {
        n115 = event-data() -> ()  [unwired: 1 in, 6 out]
        n116 = call "config_file_fgv.vi"("cmd"=enum16{"save", "load"}."load") -> ("error out"=w180:errorcluster, "var"=w179:T3)  [unwired: 8 in, 1 out]
        n117 = call "config_fgv.vi"("cmd"=enum16{"write", "read", "ini"}."write", "error in (no error)"=w180, "Config in"=w179) -> ("Config out"=w177:T3)  [unwired: 7 in, 1 out]
        n118 = local write "Config"(w177) -> ()
      }
      event "정지": Value Change {
        n119 = event-data() -> ()  [unwired: 1 in, 6 out]
        n120 = call "stop_fgv.vi"("cmd"=enum16{"default", "ini", "stop"}."stop") -> ("error out"=w182:errorcluster)  [unwired: 9 in, 1 out]
        n121 = call "Cam_Q.vi"("cmd"=enum16{"create", "write", "read", "close"}."write", "error in"=w182, "data"=enum16{"ini", "grab", "close"}."close") -> ()  [unwired: 7 in, 2 out]
        n122 = call "Strain_Q.vi"("cmd"=enum16{"create", "write", "read", "close"}."write", "error in"=w182, "data"=enum16{"run", "stop", "close"}."stop") -> ()  [unwired: 7 in, 2 out]
      }
      event "pause": Value Change {
        n123 = event-data() -> ()  [unwired: 1 in, 6 out]
        n124 = call "stop_fgv.vi"("cmd"=enum16{"default", "ini", "stop"}."stop") -> ()  [unwired: 9 in, 2 out]
      }
    }
  }
  n125 = flat-sequence {
    tunnel: w3 -> [_]
    frame #0 {
      n126 = call "Strain_Q.vi"("cmd"=enum16{"create", "write", "read", "close"}."close") -> ()  [unwired: 9 in, 2 out]
      n127 = call "Q_daq-data.vi"("cmd"=enum16{"create", "wirte", "read", "close"}."close") -> ()  [unwired: 9 in, 2 out]
      n128 = call "Cam_Q.vi"("cmd"=enum16{"create", "write", "read", "close"}."close") -> ()  [unwired: 9 in, 2 out]
    }
  }
